vi "3-Sine Wave Graph (while loop).vi"() -> ()   [LabVIEW 2014]
doc: "Sine Wave Graphy (While Loop)\nTextbook 3.11"
panel:
  out "Array":dbl[](array[numeric])
  out "Waveform Graph":cluster{i32, dbl, dbl[]}(graph)
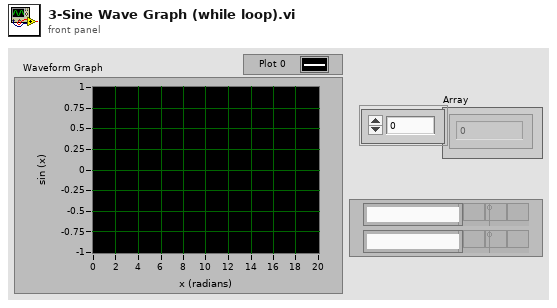
[diagram p1: front panel]
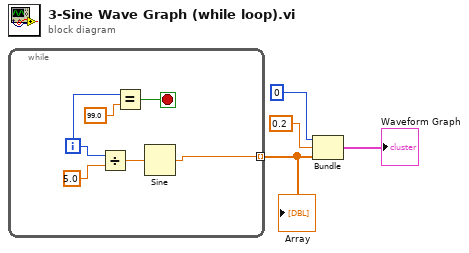
[diagram p0: block diagram]
diagram:
  n1 = while {
    tunnel: [w5] -> w1 mode=indexing
    i -> [w7]
    stop <- w6 stop-if-true
    n2 = Divide(x=w7, y=5.0) -> (x/y=w10:dbl)
    n3 = Equal?(x=w7, y=99.0) -> (x = y?=w6:bool)
    n4 = Sine(x=w10) -> (sin(x)=w5:dbl)
  }
  "Array" <- w1
  n5 = Bundle(0, 0.2, w1) -> (→"Waveform Graph":cluster{i32, dbl, dbl[]})  [unwired: 1 in]
